vi "getAlias.vi"(8 "error in (no error)":errorcluster, 10 "Topic":string, 11 "DICT in":refnum<class "DICT.lvclass">) -> (0 "error out":errorcluster, 2 "Alias":string, 3 "DICT out":refnum<class "DICT.lvclass">)   [LabVIEW 2017, in "DICT.lvclass"]
uses:
  DICT.lvclass
  DICT.lvclass/DICT.ctl
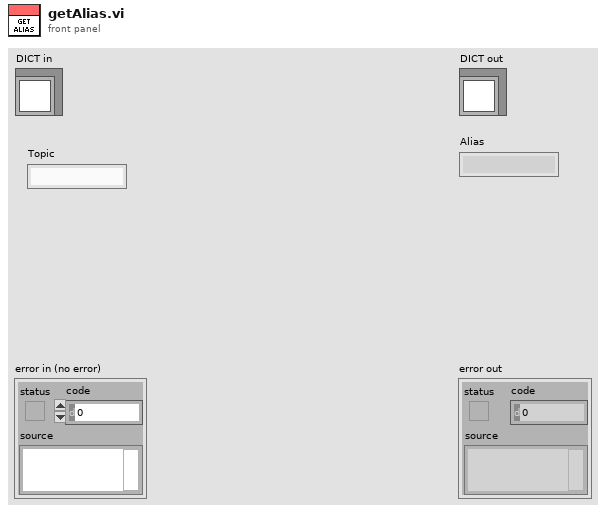
[diagram p1: front panel]
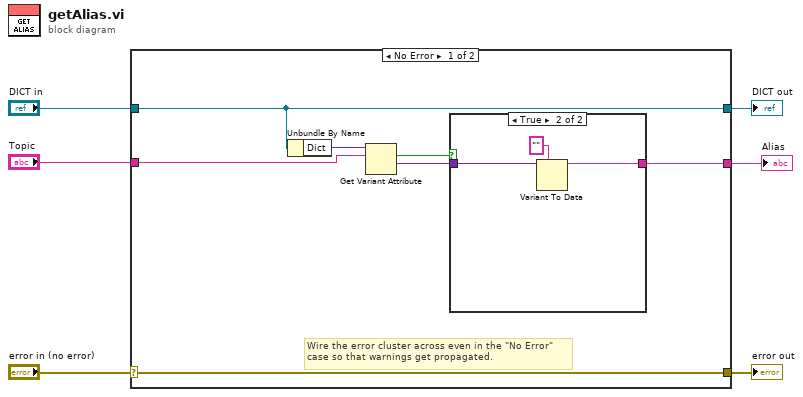
[diagram p0: block diagram]
diagram:
  n1 = case shown="No Error" "error in (no error)" {
    selector: "error in (no error)" -> [w13 w18]
    tunnel: [w13 w18] -> w5
    tunnel: [w12 w17] -> w3
    tunnel: "DICT in" -> [w12 w17]
    tunnel: "Topic" -> [w10 _]
    tunnel: [w8 _] -> w1
    frame No Error {
      # "Wire the error cluster across even in the \"No Error\"\ncase so that warnings get propagated."
      n2 = Unbundle By Name(w12) -> ("Dict"=w11:variant)
      n3 = Get Variant Attribute(Variant=w11, name=w10) -> (found=w7:bool, value=w9:variant)  [unwired: 2 in, 2 out]
      n4 = case shown="True" w7 {
        tunnel: w9 -> [_ w16]
        tunnel: [_ w14] -> w8
        frame False {
        }
        frame True {
          n5 = Variant To Data(type="" ("Topic"), Variant=w16) -> (data=w14:string)  [unwired: 1 in, 1 out]
        }
      }
    }
    frame Error {
    }
  }
  "error out" <- w5
  "DICT out" <- w3
  "Alias" <- w1
